vi "Inject Log Event.vi"(6 "timeout in ms (-1)":i32=-1, 8 "error in (no error)":errorcluster, 10 "Log Event":refnum<user-event>, 11 "NewTemplate in":refnum<class "ErrorViewer.lvclass">) -> (0 "error out":errorcluster, 1 "timed out?":bool, 3 "NewTemplate out":refnum<class "ErrorViewer.lvclass">)   [LabVIEW 2024, in "ErrorViewer.lvclass"]
uses:
  ErrorViewer.lvclass
  ErrorViewer.lvclass/ErrorViewer.ctl
  C:/Git/JA/JQMH/RQMHCore/ModuleCore/Module.lvclass
  C:/Git/JA/JQMH/ModuleTemplates/ErrorViewer/ErrorViewer.lvclass
  RQMHCore/ModuleCore/Module.lvclass
  RQMHCore/ModuleCore/Reply.ctl
  RQMHCore/ErrorReporting/Record/LogRecord.lvclass
  InjectLogEvent.ctl
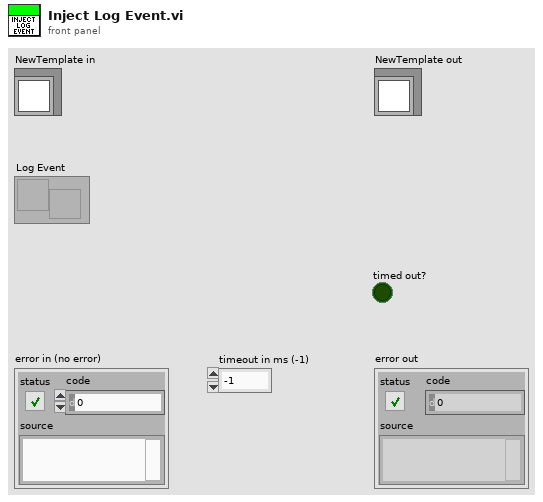
[diagram p1: front panel]
types:
  T1 = typedef "ErrorViewer.lvclass/InjectLogEvent.ctl" = cluster{"Log Event":refnum<user-event>}
  T2 = typedef "Module.lvclass/Reply.ctl" = cluster{"Expects Reply":bool, "Reply":refnum<notifier>}
  T3 = cluster{"reply":variant, "error in (no error)":errorcluster}
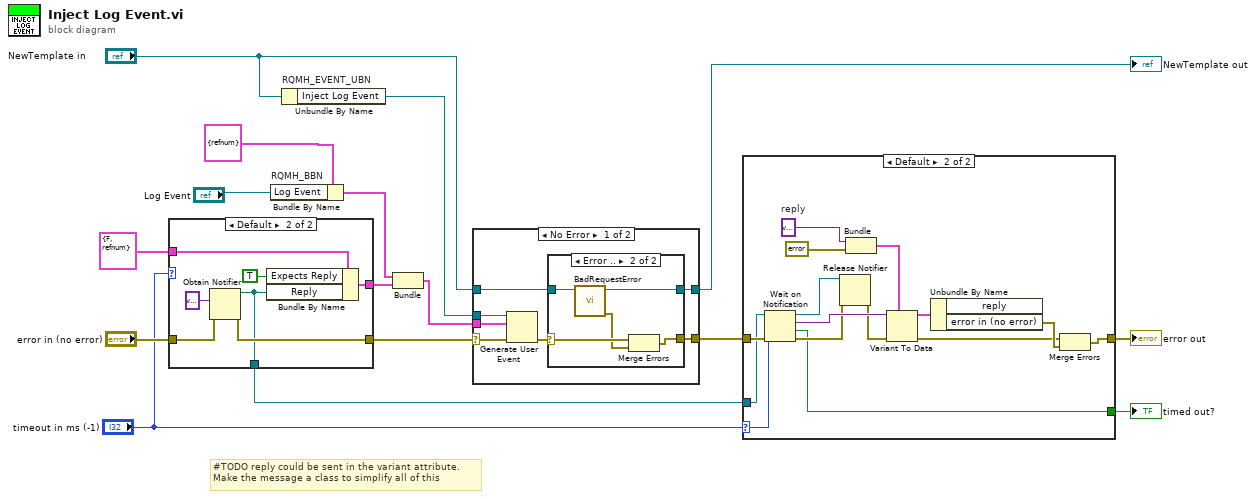
[diagram p0: block diagram]
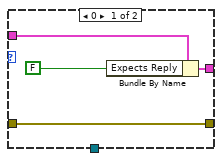
[diagram p4: hidden frame]
diagram:
  # "#TODO reply could be sent in the variant attribute.\nMake the message a class to simplify all of this"
  n1 = case shown="Default" "timeout in ms (-1)" {
    tunnel: [w19 w26] -> w12
    tunnel: "error in (no error)" -> [w17 w25]
    tunnel: [w17 w24] -> w9
    tunnel: [_ w23] -> w7
    tunnel: T2 {"Expects Reply"=FALSE, "Reply"=refnum} ("Reply") -> [w20 w22]
    frame 0 {
      n2 = Bundle By Name(cluster=w20, "Expects Reply"=FALSE) -> (w19:T2)
    }
    frame Default {
      n3 = Obtain Notifier(notification data type=variant, error in (no error)=w25) -> (notifier out=w23:refnum<notifier>, error out=w24:errorcluster)  [unwired: 2 in, 1 out]
      n4 = Bundle By Name(cluster=w22, "Expects Reply"=TRUE, "Reply"=w23) -> (w26:T2)
    }
  }
  n5 = Bundle By Name "RQMH_BBN"(cluster=T1 {"Log Event"=refnum} ("Args"), "Log Event"="Log Event") -> (w13:T1)
  n6 = Unbundle By Name "RQMH_EVENT_UBN"("NewTemplate in") -> ("Inject Log Event"=w16:refnum<user-event>)
  n7 = Bundle("Args"=w13, "Reply"=w12) -> (w11:cluster{"Args":T1, "Reply":T2})  [unwired: 1 in]
  n8 = case shown="No Error" w9 {
    selector: w9 -> [w32 w42]
    tunnel: w11 -> [w28 _]
    tunnel: w16 -> [w34 _]
    tunnel: [w31 w42] -> w8
    tunnel: "NewTemplate in" -> [w30 w43]
    tunnel: [w29 w43] -> w14
    frame No Error {
      n9 = Generate User Event(user event=w34, event data cluster=w28, error in=w32) -> (error out=w33:errorcluster)  [unwired: 1 in, 1 out]
      n10 = case shown="Error .." w33 {
        selector: w33 -> [w35 w41]
        tunnel: [w35 w40] -> w31
        tunnel: w30 -> [w36 w39]
        tunnel: [w36 w38] -> w29
        frame No Error {
        }
        frame Error {
          n11 = call "BadRequestError.vi"("JQMHModule in"=w39) -> ("error out"=w37:errorcluster, "JQMHModule out"=w38:refnum<class "ErrorViewer.lvclass">)  [unwired: 9 in]
          n12 = Merge Errors(w41, w37) -> (w40:errorcluster)
        }
      }
    }
    frame Error {
    }
  }
  "NewTemplate out" <- w14
  n13 = case shown="Default" "timeout in ms (-1)" {
    selector: "timeout in ms (-1)" -> [_ w46]
    tunnel: w8 -> [w44 w59]
    tunnel: w7 -> [_ w58]
    tunnel: [w44 w51] -> w6
    tunnel: [_ w47] -> w5
    frame 0 {
    }
    frame Default {
      w45 = variant  # reply
      n14 = Wait on Notification(notifier=w58, timeout in ms (-1)=w46, error in (no error)=w59) -> (notifier out=w50:refnum<notifier>, notification=w55:variant, timed out?=w47:bool, error out=w49:errorcluster)  [unwired: 1 in]
      n15 = Release Notifier(notifier=w50, error in (no error)=w49) -> (error out=w48:errorcluster)  [unwired: 1 in, 2 out]
      n16 = Bundle("reply"=w45, "error in (no error)"=errorcluster {"status"=FALSE, "code"=0, "source"=""}) -> (w57:T3)  [unwired: 1 in]
      n17 = Variant To Data(error in=w48, type=w57, Variant=w55) -> (data=w54:T3, error out=w52:errorcluster)
      n18 = Unbundle By Name(w54) -> ("error in (no error)"=w53:errorcluster)  [unwired: 1 out]
      n19 = Merge Errors(w52, w53) -> (w51:errorcluster)
    }
  }
  "error out" <- w6
  "timed out?" <- w5
